vi "test-Function-Generator-Matrix-Test1.vi"(8 "error in (no error)":errorcluster) -> (0 "error out":errorcluster, 3 "All tests passed":bool)   [LabVIEW 2019]
uses:
  <vilib>/Rock Robotics/WPI/ThirdParty/JAS_Junk/TrajLib/FUNCTION_GENERATOR_MATRIX.ctl
  <vilib>/Analysis/Matrix/Datatypes/RealMatrix.ctl
  <vilib>/Rock Robotics/WPI/ThirdParty/JAS_Junk/TrajLib/MatBuilder_Create.vi
  <vilib>/gmath/interp.llb/Search Ordered Table.vi
  <vilib>/Analysis/Matrix/Numeric/Add/Add (Elementwise) - RM,R.vi
  <vilib>/Rock Robotics/WPI/ThirdParty/JAS_Junk/TrajLib/Trajectory_Library.lvlib
  <vilib>/Analysis/Matrix/NI_Matrix.lvlib
panel:
  out "T 9":T1
  out "T empty":T1
  out "T 8":T1
  out "T 7":T1
  out "T 6":T1
  out "T 5":T1
  out "T 4":T1
  out "T 3":T1
  out "T 2":T1
  out "T 1":T1
  out "T 0":T1
  out "out FUNC_GEN_MATRIX":T2
  out "Table Ys":variant[](array[variant])
  out "Table Xs":dbl[](array[numeric])
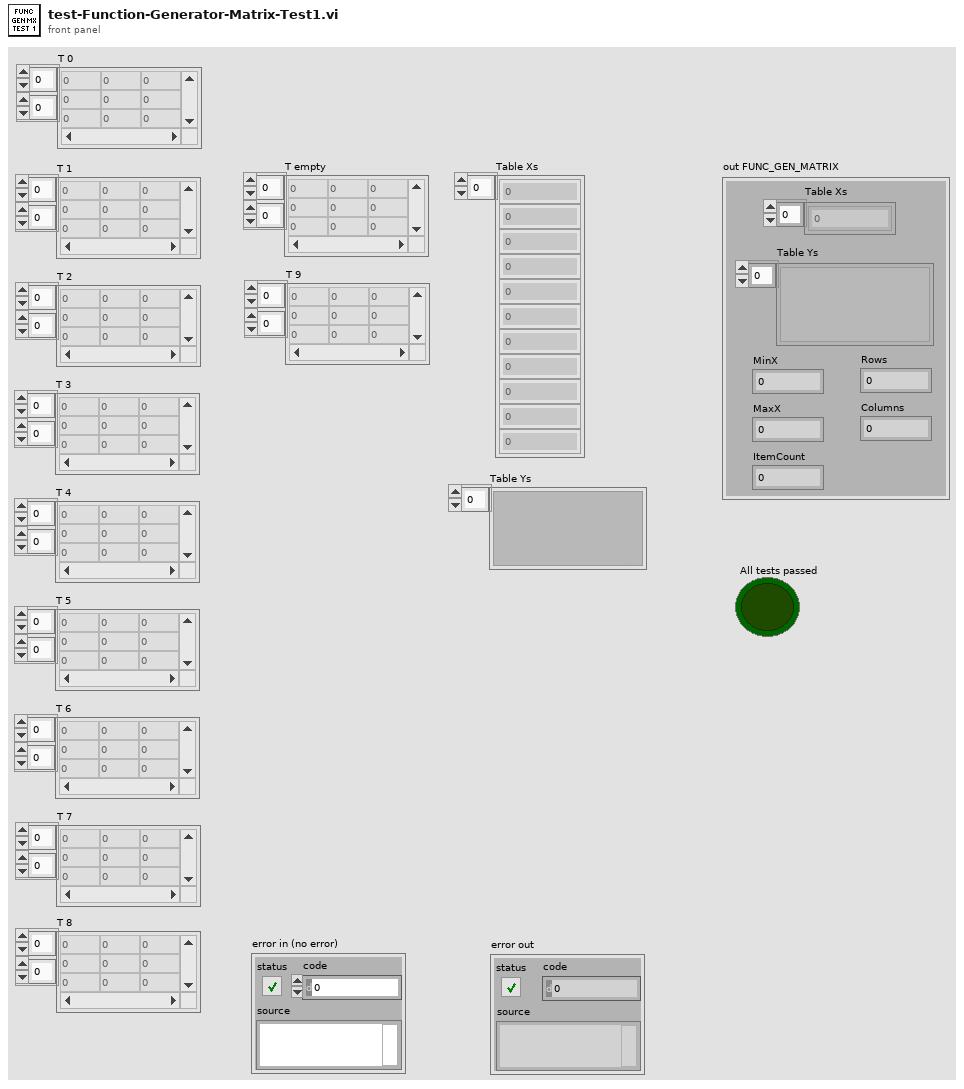
[diagram p1: front panel]
types:
  T1 = typedef "NI_Matrix.lvlib/RealMatrix.ctl" = dbl[][]
  T2 = typedef "Trajectory_Library.lvlib/FUNCTION_GENERATOR_MATRIX.ctl" = cluster{"Table Xs":dbl[], "Table Ys":variant[], "MinX":dbl, "MaxX":dbl, "ItemCount":i32, "Rows":i32, "Columns":i32}
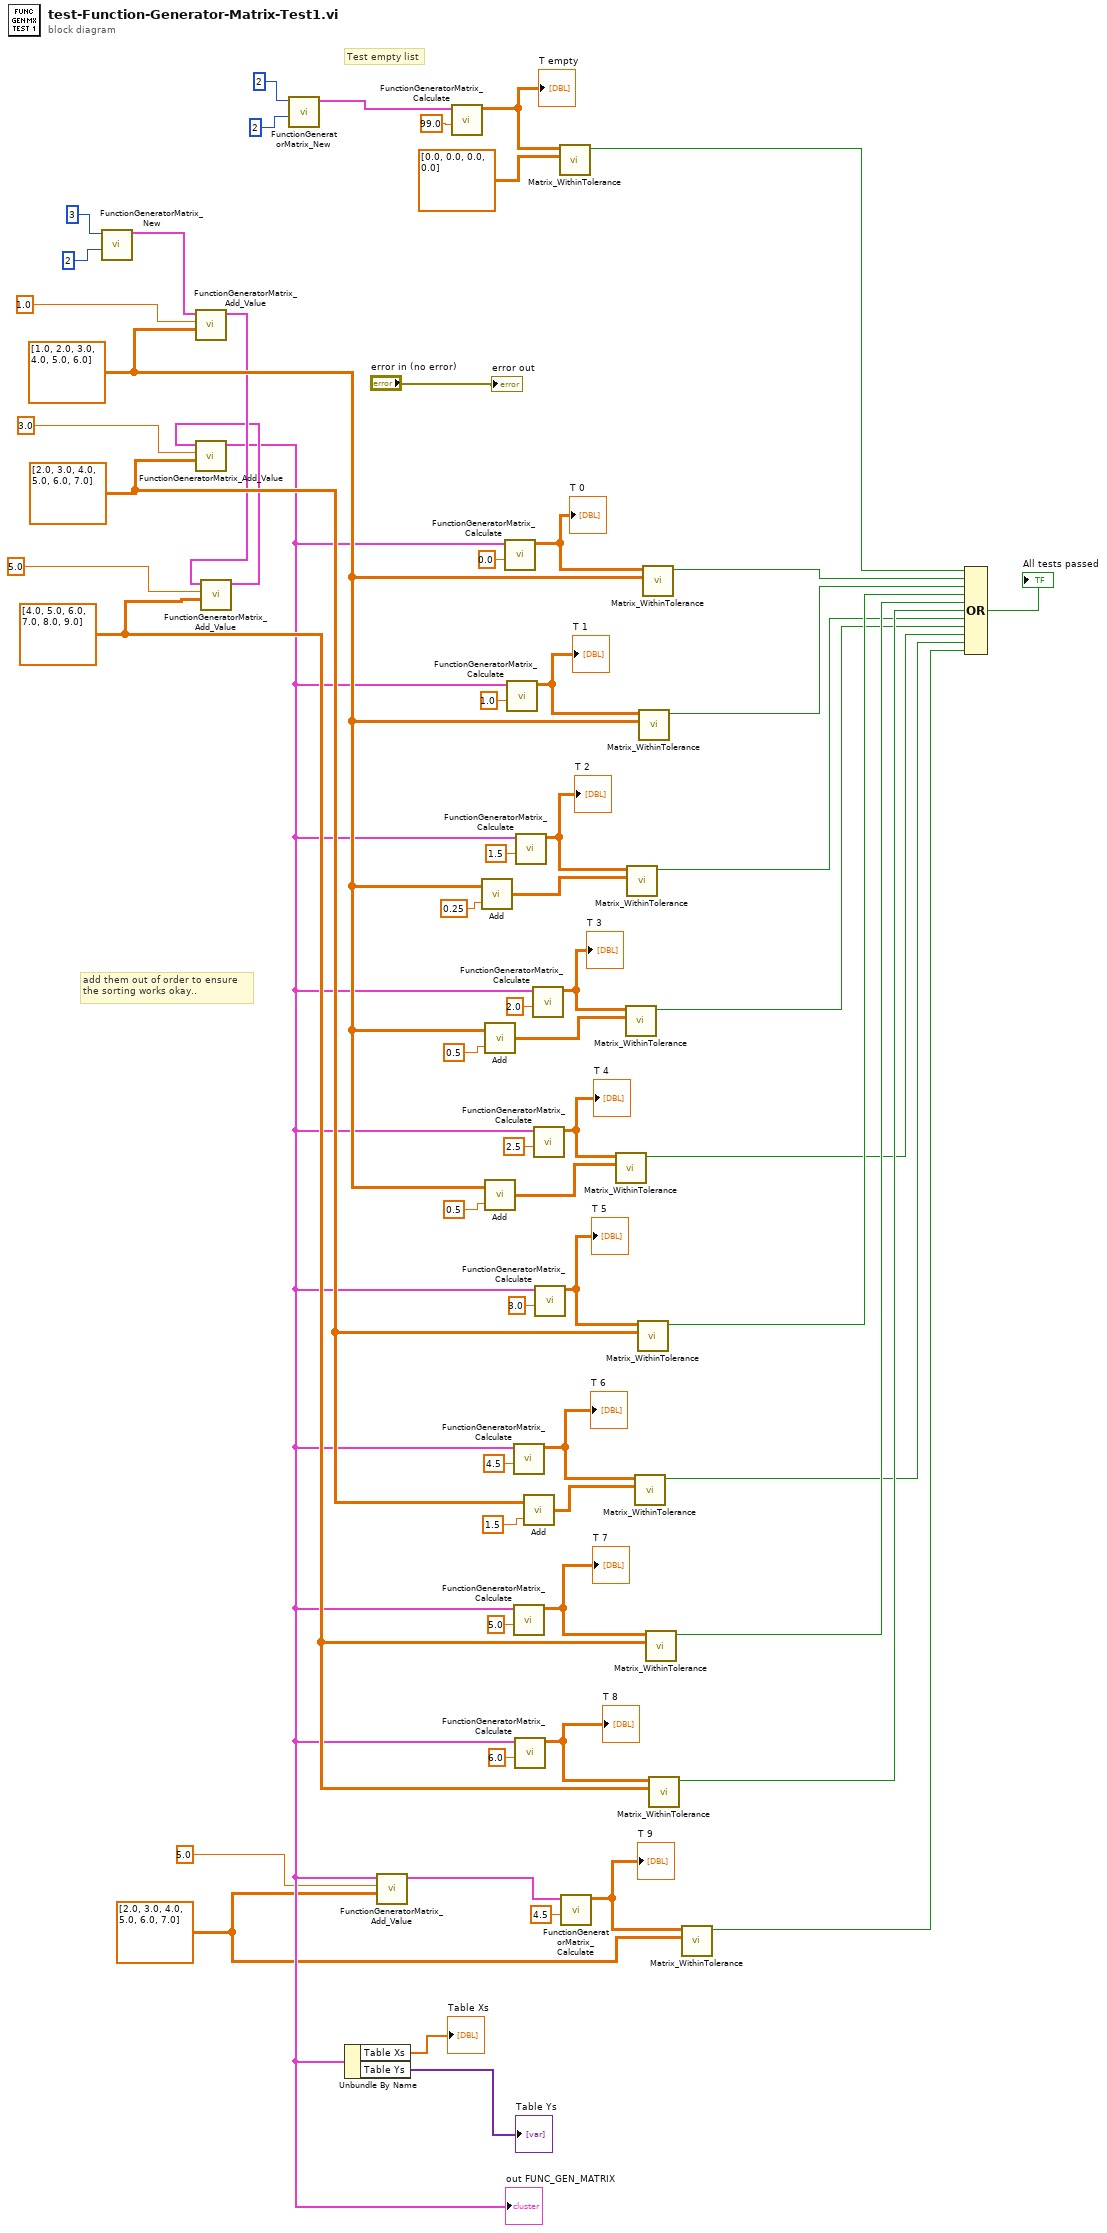
[diagram p0: block diagram]
diagram:
  w2 = T1 [[2.0, 3.0], [4.0, 5.0], [6.0, 7.0]] ("Y Value")
  w37 = T1 [[4.0, 5.0], [6.0, 7.0], [8.0, 9.0]] ("Y Value")
  w12 = T1 [[2.0, 3.0], [4.0, 5.0], [6.0, 7.0]] ("Y Value")
  w18 = T1 [[1.0, 2.0], [3.0, 4.0], [5.0, 6.0]] ("Y Value")
  # "Test empty list"
  # "add them out of order to ensure\nthe sorting works okay.."
  n1 = call <vilib>:"FunctionGeneratorMatrix_New.vi"("Columns"=2, "Rows"=3) -> ("FUNCTION_GENERATOR_MATRIX"=w60:T2)  [unwired: 9 in]
  n2 = call <vilib>:"FunctionGeneratorMatrix_Add_Value.vi"("Y Value"=w18, "X Value"=1.0, "in FUNC_GEN_MATRIX"=w60) -> ("out FUNC_GEN_MATRIX"=w9:T2)  [unwired: 7 in, 1 out]
  n3 = call <vilib>:"FunctionGeneratorMatrix_Add_Value.vi"("Y Value"=w37, "X Value"=5.0, "in FUNC_GEN_MATRIX"=w9) -> ("out FUNC_GEN_MATRIX"=w8:T2)  [unwired: 7 in, 1 out]
  n4 = call <vilib>:"FunctionGeneratorMatrix_Add_Value.vi"("Y Value"=w12, "X Value"=3.0, "in FUNC_GEN_MATRIX"=w8) -> ("out FUNC_GEN_MATRIX"=w7:T2)  [unwired: 7 in, 1 out]
  "out FUNC_GEN_MATRIX" <- w7
  n5 = call <vilib>:"FunctionGeneratorMatrix_New.vi"("Columns"=2, "Rows"=2) -> ("FUNCTION_GENERATOR_MATRIX"=w31:T2)  [unwired: 9 in]
  n6 = Unbundle By Name(w7) -> ("Table Xs"=→"Table Xs":dbl[], "Table Ys"=→"Table Ys":variant[])
  n7 = call <vilib>:"FunctionGeneratorMatrix_Add_Value.vi"("Y Value"=w2, "X Value"=5.0, "in FUNC_GEN_MATRIX"=w7) -> ("out FUNC_GEN_MATRIX"=w3:T2)  [unwired: 7 in, 1 out]
  n8 = call <vilib>:"FunctionGeneratorMatrix_Calculate.vi"("Input Value"=99.0, "FUNCTION_GENERATOR_MATRIX"=w31) -> ("Output Matrix"=w30:T1)  [unwired: 9 in]
  "T empty" <- w30
  n9 = call-poly <vilib>:"Add.vi"("Real Scalar c"=0.25, "Real Matrix A"=w18) -> ("A + c"=w25:T1)
  n10 = call-poly <vilib>:"Add.vi"("Real Scalar c"=0.5, "Real Matrix A"=w18) -> ("A + c"=w22:T1)
  n11 = call-poly <vilib>:"Add.vi"("Real Scalar c"=0.5, "Real Matrix A"=w18) -> ("A + c"=w16:T1)
  n12 = call <vilib>:"FunctionGeneratorMatrix_Calculate.vi"("Input Value"=0.0, "FUNCTION_GENERATOR_MATRIX"=w7) -> ("Output Matrix"=w46:T1)  [unwired: 9 in]
  "T 0" <- w46
  n13 = call <vilib>:"FunctionGeneratorMatrix_Calculate.vi"("Input Value"=1.0, "FUNCTION_GENERATOR_MATRIX"=w7) -> ("Output Matrix"=w45:T1)  [unwired: 9 in]
  "T 1" <- w45
  n14 = call <vilib>:"FunctionGeneratorMatrix_Calculate.vi"("Input Value"=4.5, "FUNCTION_GENERATOR_MATRIX"=w7) -> ("Output Matrix"=w13:T1)  [unwired: 9 in]
  "T 6" <- w13
  n15 = call <vilib>:"FunctionGeneratorMatrix_Calculate.vi"("Input Value"=5.0, "FUNCTION_GENERATOR_MATRIX"=w7) -> ("Output Matrix"=w41:T1)  [unwired: 9 in]
  "T 7" <- w41
  n16 = call <vilib>:"FunctionGeneratorMatrix_Calculate.vi"("Input Value"=6.0, "FUNCTION_GENERATOR_MATRIX"=w7) -> ("Output Matrix"=w40:T1)  [unwired: 9 in]
  "T 8" <- w40
  n17 = call <vilib>:"FunctionGeneratorMatrix_Calculate.vi"("Input Value"=1.5, "FUNCTION_GENERATOR_MATRIX"=w7) -> ("Output Matrix"=w26:T1)  [unwired: 9 in]
  "T 2" <- w26
  n18 = call-poly <vilib>:"Add.vi"("Real Scalar c"=1.5, "Real Matrix A"=w12) -> ("A + c"=w11:T1)
  n19 = call <vilib>:"FunctionGeneratorMatrix_Calculate.vi"("Input Value"=2.0, "FUNCTION_GENERATOR_MATRIX"=w7) -> ("Output Matrix"=w23:T1)  [unwired: 9 in]
  "T 3" <- w23
  n20 = call <vilib>:"FunctionGeneratorMatrix_Calculate.vi"("Input Value"=2.5, "FUNCTION_GENERATOR_MATRIX"=w7) -> ("Output Matrix"=w17:T1)  [unwired: 9 in]
  "T 4" <- w17
  n21 = call <vilib>:"FunctionGeneratorMatrix_Calculate.vi"("Input Value"=3.0, "FUNCTION_GENERATOR_MATRIX"=w7) -> ("Output Matrix"=w39:T1)  [unwired: 9 in]
  "T 5" <- w39
  n22 = call <vilib>:"Matrix_WithinTolerance.vi"("Matrix B"=T1 [[0.0, 0.0], [0.0, 0.0]] ("Y Value"), "Matrix A"=w30) -> ("WithinTolerance"=w28:bool)  [unwired: 8 in, 1 out]
  n23 = call <vilib>:"FunctionGeneratorMatrix_Calculate.vi"("Input Value"=4.5, "FUNCTION_GENERATOR_MATRIX"=w3) -> ("Output Matrix"=w4:T1)  [unwired: 9 in]
  "T 9" <- w4
  n24 = call <vilib>:"Matrix_WithinTolerance.vi"("Matrix B"=w16, "Matrix A"=w17) -> ("WithinTolerance"=w15:bool)  [unwired: 8 in, 1 out]
  n25 = call <vilib>:"Matrix_WithinTolerance.vi"("Matrix B"=w22, "Matrix A"=w23) -> ("WithinTolerance"=w20:bool)  [unwired: 8 in, 1 out]
  n26 = call <vilib>:"Matrix_WithinTolerance.vi"("Matrix B"=w25, "Matrix A"=w26) -> ("WithinTolerance"=w21:bool)  [unwired: 8 in, 1 out]
  n27 = call <vilib>:"Matrix_WithinTolerance.vi"("Matrix B"=w11, "Matrix A"=w13) -> ("WithinTolerance"=w10:bool)  [unwired: 8 in, 1 out]
  n28 = call <vilib>:"Matrix_WithinTolerance.vi"("Matrix B"=w12, "Matrix A"=w39) -> ("WithinTolerance"=w38:bool)  [unwired: 8 in, 1 out]
  n29 = call <vilib>:"Matrix_WithinTolerance.vi"("Matrix B"=w18, "Matrix A"=w45) -> ("WithinTolerance"=w42:bool)  [unwired: 8 in, 1 out]
  n30 = call <vilib>:"Matrix_WithinTolerance.vi"("Matrix B"=w18, "Matrix A"=w46) -> ("WithinTolerance"=w44:bool)  [unwired: 8 in, 1 out]
  n31 = call <vilib>:"Matrix_WithinTolerance.vi"("Matrix B"=w37, "Matrix A"=w41) -> ("WithinTolerance"=w36:bool)  [unwired: 8 in, 1 out]
  n32 = call <vilib>:"Matrix_WithinTolerance.vi"("Matrix B"=w37, "Matrix A"=w40) -> ("WithinTolerance"=w35:bool)  [unwired: 8 in, 1 out]
  n33 = call <vilib>:"Matrix_WithinTolerance.vi"("Matrix B"=w2, "Matrix A"=w4) -> ("WithinTolerance"=w1:bool)  [unwired: 8 in, 1 out]
  n34 = Compound Arithmetic op=OR(w28, w44, w42, w38, w36, w35, w21, w20, w15, w10, w1) -> (→"All tests passed":bool)
  "error out" <- "error in (no error)"
